vi "MCLB_AssertIndexValue_Tests.vi"(11 "error in":errorcluster) -> (15 "error out":errorcluster)   [LabVIEW 2016, in "DronaTest.lvlib"]
uses:
  DronaTest.lvlib
  APIs/Stimulus/ControlValue/SetValueAuto.vi
  APIs/Assert/AssertControlValue/Controls/MC Listbox/AssertIndexValue.vi
  <vilib>/addons/_JKI Toolkits/Caraya/classes/Assert/Assert Error.vi
  <vilib>/addons/_JKI Toolkits/Caraya/classes/Assert/Assert Equal Value_Variant.vi
  <vilib>/addons/_JKI Toolkits/Caraya/classes/Test/Test.lvclass
  Drona.lvlib
  <vilib>/SLL Toolkit/SLL Debug/SLL Debug.lvlib
  <vilib>/addons/_JKI Toolkits/Caraya/classes/Assert/Assert.lvclass
  APIs/Assert/AssertControlValue/Controls/MC Listbox/AssertMCListbox.lvlib
  APIs/Stimulus/ControlValue/ControlValue.lvlib
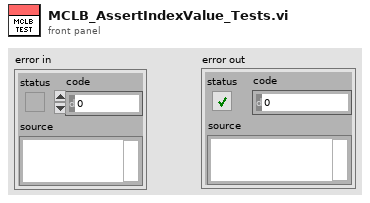
[diagram p1: front panel]
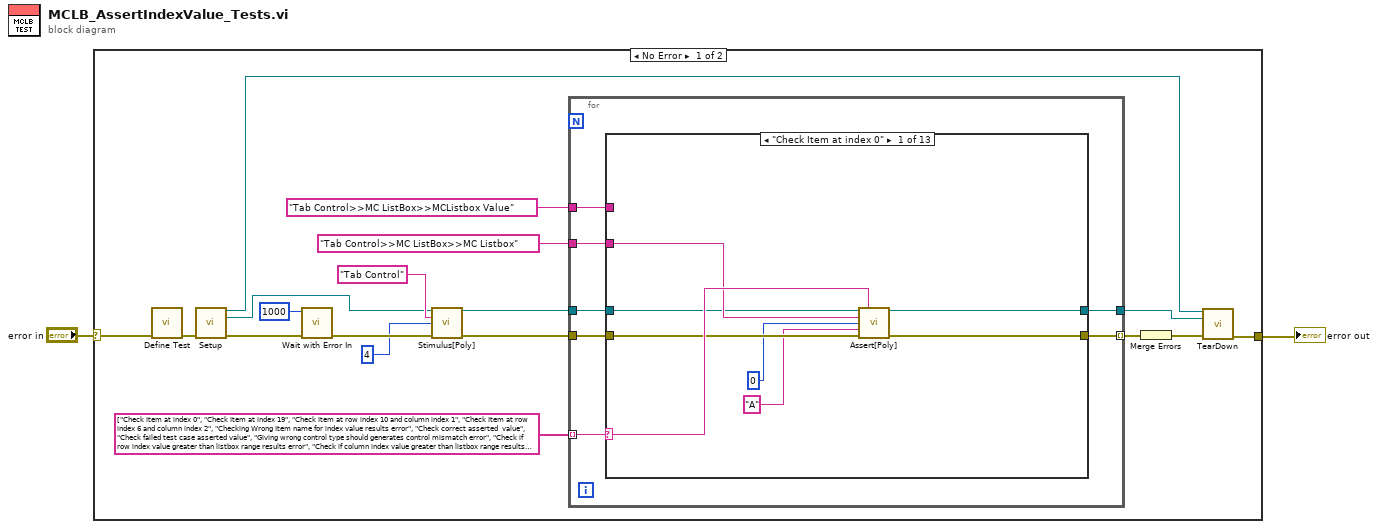
[diagram p0: block diagram]
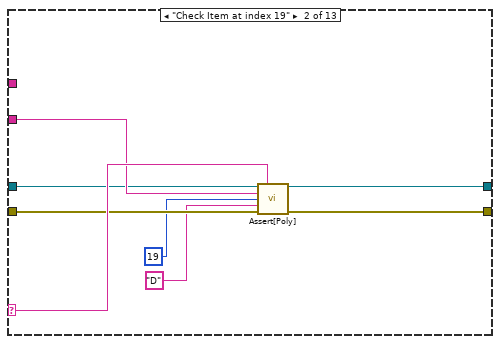
[diagram p2: hidden frame]
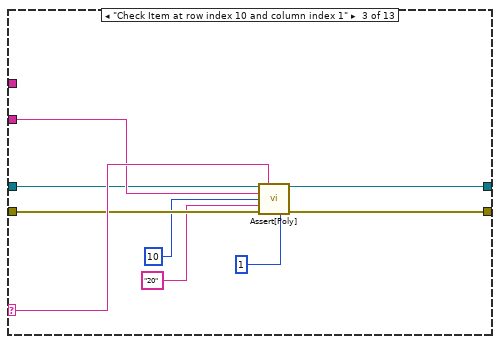
[diagram p3: hidden frame]
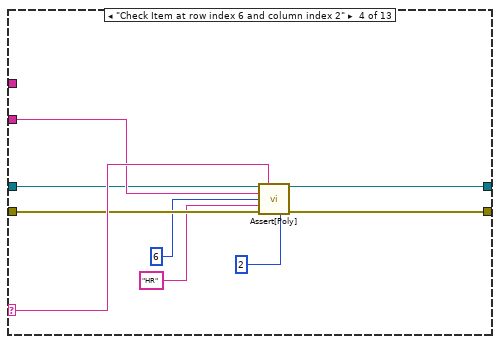
[diagram p4: hidden frame]
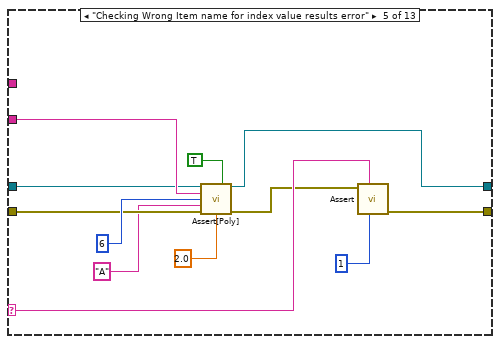
[diagram p5: hidden frame]
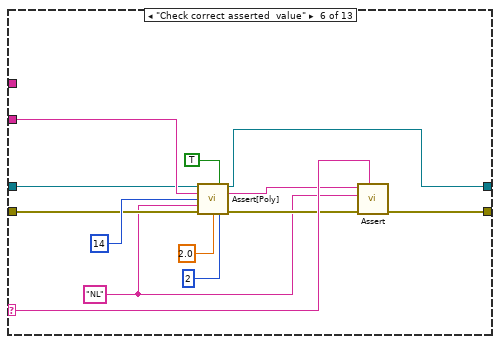
[diagram p6: hidden frame]
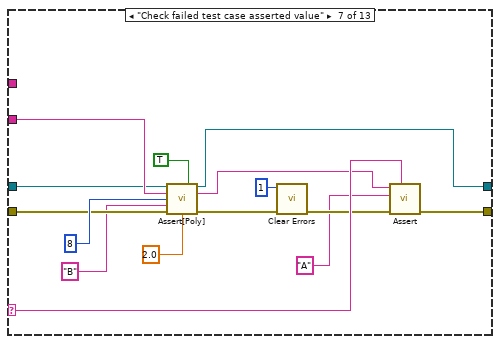
[diagram p7: hidden frame]
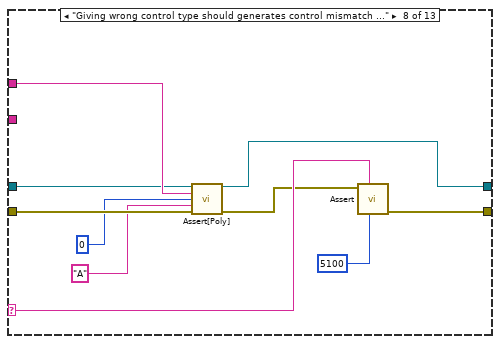
[diagram p8: hidden frame]
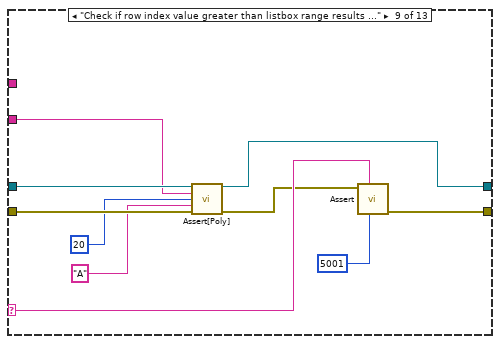
[diagram p9: hidden frame]
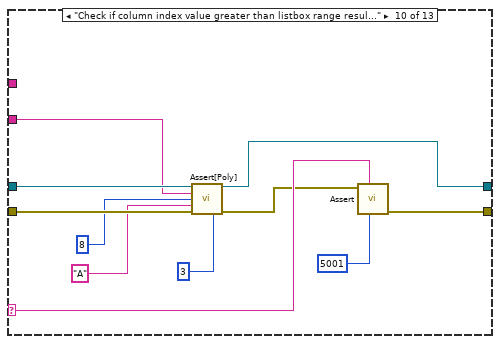
[diagram p10: hidden frame]
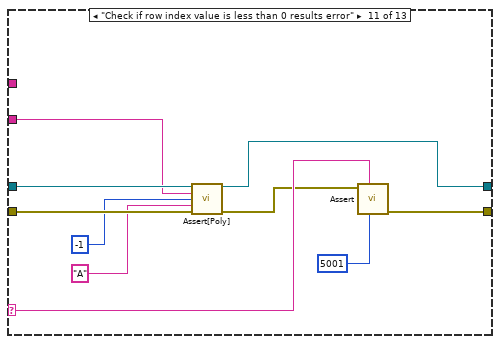
[diagram p11: hidden frame]
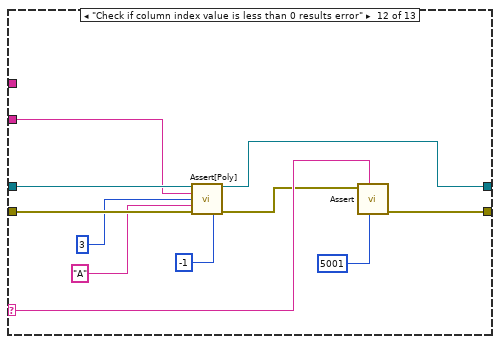
[diagram p12: hidden frame]
diagram:
  n1 = case shown="No Error" "error in" {
    selector: "error in" -> [w20 w156]
    tunnel: [w3 w156] -> w1
    frame No Error {
      n2 = call <vilib>:"Define Test.vi"("error in (no error)"=w20) -> ("error out"=w9:errorcluster)  [unwired: 9 in, 1 out]
      n3 = call "Setup.vi"("error in"=w9) -> ("Application Ref"=w5:refnum<vi>, "VI out"=w7:refnum<vi>, "error out"=w8:errorcluster)  [unwired: 12 in]
      n4 = call <vilib>:"Wait with Error In.vi"("error in (no error)"=w8, "milliseconds to wait"=u32 1000) -> ("error out"=w18:errorcluster)  [unwired: 9 in]
      n5 = call-poly "Stimulus[Poly].vi"("VI Reference In"=w7, "Control Path"="Tab Control", "Value (Signaling)"=4, "error in"=w18) -> ("VI Reference Out"=w14:refnum<vi>, "error out"=w17:errorcluster)  [unwired: 10 in]
      n6 = for {
        tunnel: w14 -> [w26]
        tunnel: "Tab Control>>MC ListBox>>MC Listbox" ("Control Path") -> [w25]
        tunnel: "Tab Control>>MC ListBox>>MCListbox Value" ("Control Path") -> [w24]
        tunnel: string[] ["Check Item at index 0", "Check Item at index 19", "Check Item at row index 10 and column index 1", "Check Item at row index 6 and column index 2", "Checking Wrong Item name for index value results error", "Check correct asserted  value", "Check failed test case asserted value", "Giving wrong control type should generates control mismatch error", "Check if row index value greater than listbox range results error", "Check if column index value greater than listbox range results error", "Check if row index value is less than 0 results error", "Check if column index value is less than 0 results error"] -> [w22] mode=indexing
        tunnel: [w21] -> w4
        tunnel: w17 -> [w27]
        tunnel: [w23] -> w10 mode=indexing
        n7 = case shown="\"Check Item at index 0\"" w22 {
          selector: w22 -> [w33 w41 w50 w59 w72 w85 w100 w110 w120 w131 w141 w152 _]
          tunnel: w27 -> [w31 w39 w48 w57 w64 w80 w95 w105 w116 w127 w137 w148 w155]
          tunnel: w26 -> [w30 w38 w47 w56 w63 w79 w94 w104 w115 w126 w136 w147 w154]
          tunnel: w25 -> [w32 w40 w49 w58 w70 w84 w99 _ w112 w123 w133 w144 _]
          tunnel: w24 -> [_ _ _ _ _ _ _ w107 _ _ _ _ _]
          tunnel: [w35 w43 w52 w61 w73 w86 w101 w111 w121 w132 w142 w153 w155] -> w23
          tunnel: [w34 w42 w51 w60 w68 w82 w97 w106 w117 w128 w138 w149 w154] -> w21
          frame "Check Item at index 0" {
            n8 = call-poly "Assert[Poly].vi"("VI Reference In"=w30, "Test Label"=w33, "Control Path"=w32, "Row Index"=0 ("Item Index"), "Item Value"="A", "Error In"=w31) -> ("VI Reference Out"=w34:refnum<vi>, "Error Out"=w35:errorcluster)  [unwired: 7 in, 1 out]
          }
          frame "Check Item at index 19" {
            n9 = call-poly "Assert[Poly].vi"("VI Reference In"=w38, "Test Label"=w41, "Control Path"=w40, "Row Index"=19 ("Item Index"), "Item Value"="D", "Error In"=w39) -> ("VI Reference Out"=w42:refnum<vi>, "Error Out"=w43:errorcluster)  [unwired: 7 in, 1 out]
          }
          frame "Check Item at row index 10 and column index 1" {
            n10 = call-poly "Assert[Poly].vi"("VI Reference In"=w47, "Test Label"=w50, "Control Path"=w49, "Row Index"=10 ("Item Index"), "Item Value"="20", "Error In"=w48, "Column Index"=1) -> ("VI Reference Out"=w51:refnum<vi>, "Error Out"=w52:errorcluster)  [unwired: 6 in, 1 out]
          }
          frame "Check Item at row index 6 and column index 2" {
            n11 = call-poly "Assert[Poly].vi"("VI Reference In"=w56, "Test Label"=w59, "Control Path"=w58, "Row Index"=6 ("Item Index"), "Item Value"="HR", "Error In"=w57, "Column Index"=2) -> ("VI Reference Out"=w60:refnum<vi>, "Error Out"=w61:errorcluster)  [unwired: 6 in, 1 out]
          }
          frame "Checking Wrong Item name for index value results error" {
            n12 = call-poly "Assert[Poly].vi"("VI Reference In"=w63, "Assert Only? (F)"=TRUE, "Control Path"=w70, "Row Index"=6 ("Item Index"), "Item Value"="A", "Error In"=w64, "Timeout(5 sec)"=2.0) -> ("VI Reference Out"=w68:refnum<vi>, "Error Out"=w67:errorcluster)  [unwired: 6 in, 1 out]
            n13 = call-poly <vilib>:"Assert.vi"("error code (1)"=1, "Label"=w72, "Error?"=w67) -> ("error out"=w73:errorcluster)  [unwired: 7 in, 1 out]
          }
          frame "Check correct asserted  value" {
            w76 = "NL" ("Item Value")
            n14 = call-poly "Assert[Poly].vi"("VI Reference In"=w79, "Assert Only? (F)"=TRUE, "Control Path"=w84, "Row Index"=14 ("Item Index"), "Item Value"=w76, "Error In"=w80, "Timeout(5 sec)"=2.0, "Column Index"=2) -> ("VI Reference Out"=w82:refnum<vi>, "Asserted Value"=w77:string, "Error Out"=w78:errorcluster)  [unwired: 5 in]
            n15 = call-poly <vilib>:"Assert.vi"("Label"=w85, "error in (no error)"=w78, "Y"=w76, "X"=w77) -> ("error out"=w86:errorcluster)  [unwired: 6 in, 1 out]
          }
          frame "Check failed test case asserted value" {
            n16 = call-poly "Assert[Poly].vi"("VI Reference In"=w94, "Assert Only? (F)"=TRUE, "Control Path"=w99, "Row Index"=8 ("Item Index"), "Item Value"="B", "Error In"=w95, "Timeout(5 sec)"=2.0) -> ("VI Reference Out"=w97:refnum<vi>, "Asserted Value"=w92:string, "Error Out"=w93:errorcluster)  [unwired: 6 in]
            n17 = call <vilib>:"Clear Errors.vi"("error in (no error)"=w93, "specific error code to clear (0: all)"=1) -> ("error out"=w90:errorcluster)  [unwired: 4 in, 1 out]
            n18 = call-poly <vilib>:"Assert.vi"("Label"=w100, "error in (no error)"=w90, "Y"="A" ("Item Value"), "X"=w92) -> ("error out"=w101:errorcluster)  [unwired: 6 in, 1 out]
          }
          frame "Giving wrong control type should generates control mismatch error" {
            n19 = call-poly "Assert[Poly].vi"("VI Reference In"=w104, "Control Path"=w107, "Row Index"=0 ("Item Index"), "Item Value"="A", "Error In"=w105) -> ("VI Reference Out"=w106:refnum<vi>, "Error Out"=w108:errorcluster)  [unwired: 8 in, 1 out]
            n20 = call-poly <vilib>:"Assert.vi"("error code (1)"=5100, "Label"=w110, "Error?"=w108) -> ("error out"=w111:errorcluster)  [unwired: 7 in, 1 out]
          }
          frame "Check if row index value greater than listbox range results error" {
            n21 = call-poly "Assert[Poly].vi"("VI Reference In"=w115, "Control Path"=w112, "Row Index"=20 ("Item Index"), "Item Value"="A", "Error In"=w116) -> ("VI Reference Out"=w117:refnum<vi>, "Error Out"=w118:errorcluster)  [unwired: 8 in, 1 out]
            n22 = call-poly <vilib>:"Assert.vi"("error code (1)"=5001, "Label"=w120, "Error?"=w118) -> ("error out"=w121:errorcluster)  [unwired: 7 in, 1 out]
          }
          frame "Check if column index value greater than listbox range results error" {
            n23 = call-poly "Assert[Poly].vi"("VI Reference In"=w126, "Control Path"=w123, "Row Index"=8 ("Item Index"), "Item Value"="A", "Error In"=w127, "Column Index"=3) -> ("VI Reference Out"=w128:refnum<vi>, "Error Out"=w129:errorcluster)  [unwired: 7 in, 1 out]
            n24 = call-poly <vilib>:"Assert.vi"("error code (1)"=5001, "Label"=w131, "Error?"=w129) -> ("error out"=w132:errorcluster)  [unwired: 7 in, 1 out]
          }
          frame "Check if row index value is less than 0 results error" {
            n25 = call-poly "Assert[Poly].vi"("VI Reference In"=w136, "Control Path"=w133, "Row Index"=-1 ("Item Index"), "Item Value"="A", "Error In"=w137) -> ("VI Reference Out"=w138:refnum<vi>, "Error Out"=w139:errorcluster)  [unwired: 8 in, 1 out]
            n26 = call-poly <vilib>:"Assert.vi"("error code (1)"=5001, "Label"=w141, "Error?"=w139) -> ("error out"=w142:errorcluster)  [unwired: 7 in, 1 out]
          }
          frame "Check if column index value is less than 0 results error" {
            n27 = call-poly "Assert[Poly].vi"("VI Reference In"=w147, "Control Path"=w144, "Row Index"=3 ("Item Index"), "Item Value"="A", "Error In"=w148, "Column Index"=-1) -> ("VI Reference Out"=w149:refnum<vi>, "Error Out"=w150:errorcluster)  [unwired: 7 in, 1 out]
            n28 = call-poly <vilib>:"Assert.vi"("error code (1)"=5001, "Label"=w152, "Error?"=w150) -> ("error out"=w153:errorcluster)  [unwired: 7 in, 1 out]
          }
          frame Default {
          }
        }
      }
      n29 = Merge Errors(w10) -> (w6:errorcluster)
      n30 = call "TearDown.vi"("Application Ref"=w5, "VI in"=w4, "error in (no error)"=w6) -> ("error out"=w3:errorcluster)  [unwired: 12 in]
    }
    frame Error {
    }
  }
  "error out" <- w1
